vi "SETPINSTATUS.vi"(0 "Arduino in":refnum<class "Arduino.lvclass">, 5 "PORT":dbl, 7 "PIN":dbl, 9 "valor":bool, 11 "error in (no error)":errorcluster) -> (4 "Arduino out":refnum<class "Arduino.lvclass">, 15 "error out":errorcluster)   [LabVIEW 2019, in "Arduino.lvclass"]
uses:
  Arduino.lvclass
  Arduino.lvclass/Arduino.ctl
  37a8346b-4194-4e07-ad39-aa8e368091c5.vi
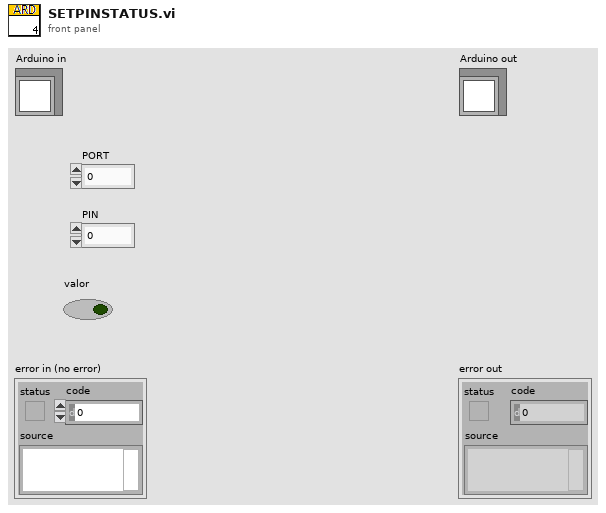
[diagram p1: front panel]
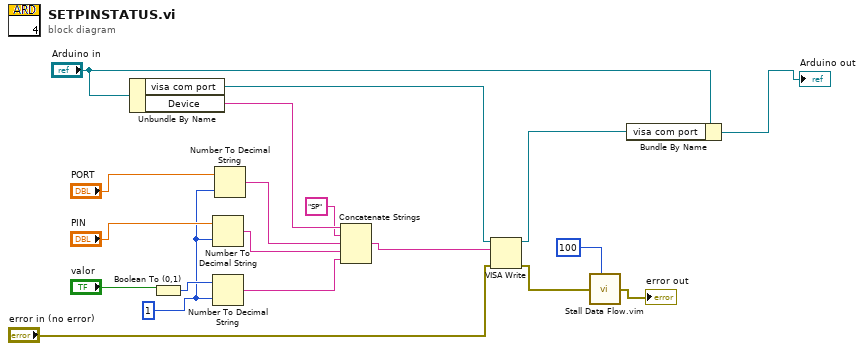
[diagram p0: block diagram]
diagram:
  w15 = i16 1 ("width (-)")
  n1 = Unbundle By Name("Arduino in") -> ("visa com port"=w14:refnum<visa-resource-name>, "Device"=w13:string)
  n2 = Boolean To (0,1)(Boolean="valor") -> (0, 1=w16:i16)
  n3 = Number To Decimal String(number="PIN", width (-)=w15) -> (decimal integer string=w10:string)
  n4 = Number To Decimal String(number=w16, width (-)=w15) -> (decimal integer string=w9:string)
  n5 = Number To Decimal String(number="PORT", width (-)=w15) -> (decimal integer string=w11:string)
  n6 = Concatenate Strings(w13, "SP" ("string"), w11, w10, w9) -> (w8:string)
  n7 = VISA Write(VISA resource name=w14, write buffer=w8, error in (no error)="error in (no error)") -> (VISA resource name out=w1:refnum<visa-resource-name>, error out=w6:errorcluster)  [unwired: 1 out]
  n8 = call "Stall Data Flow.vim"("value in"=w6, "milliseconds to wait"=u32 100) -> ("value out"=→"error out":errorcluster)  [unwired: 1 out]
  n9 = Bundle By Name(cluster="Arduino in", "visa com port"=w1) -> (→"Arduino out":refnum<class "Arduino.lvclass">)
